vi "记录个数.vi"(8 "索引字符串":string, 11 "原始数据输入":string[](array[string])) -> (3 "结果个数输出":dbl)   [LabVIEW 2011]
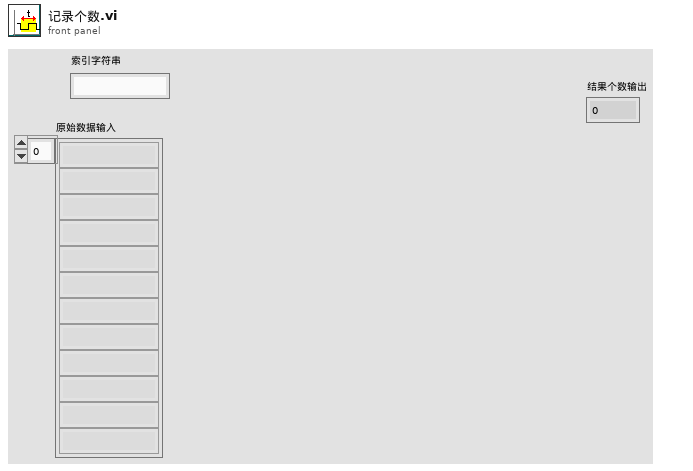
[diagram p1: front panel]
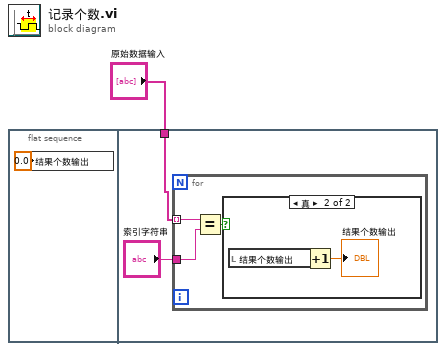
[diagram p0: block diagram]
diagram:
  n1 = flat-sequence {
    tunnel: "原始数据输入" -> [w3]
    frame #0 {
      n2 = local write "结果个数输出"(0.0 ("数值")) -> ()
    }
    frame #1 {
      n3 = for {
        tunnel: w3 -> [w7] mode=indexing
        tunnel: "索引字符串" -> [w6]
        n4 = Equal?(x=w7, y=w6) -> (x = y?=w5:bool)
        n5 = case shown="真" w5 {
          frame False {
          }
          frame True {
            n6 = local read "结果个数输出"() -> (w9:dbl)
            n7 = Increment(x=w9) -> (x+1=→"结果个数输出":dbl)
          }
        }
      }
    }
  }
